vi "Decide next action (polarization-based).vi"(8 "error in (no error)":errorcluster, 10 "Seek positive polarization?":bool, 11 "Automatic Mode in":refnum<class "Automatic Mode.lvclass">) -> (0 "error out":errorcluster, 2 "Decision":T1, 3 "Automatic Mode out":refnum<class "Automatic Mode.lvclass">)   [LabVIEW 2015, in "Automatic Mode.lvclass"]
uses:
  Automatic Mode.lvclass
  Controller decision.ctl
  Automatic Mode.lvclass/Automatic Mode.ctl
  <vilib>/gmath/NI_Gmath.lvlib
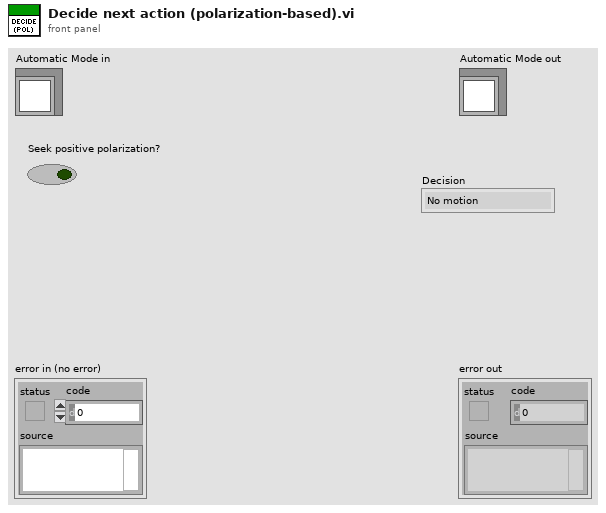
[diagram p1: front panel]
types:
  T1 = typedef "Controller decision.ctl" = enum16{"No motion", "Switch direction", "Keep current direction"}
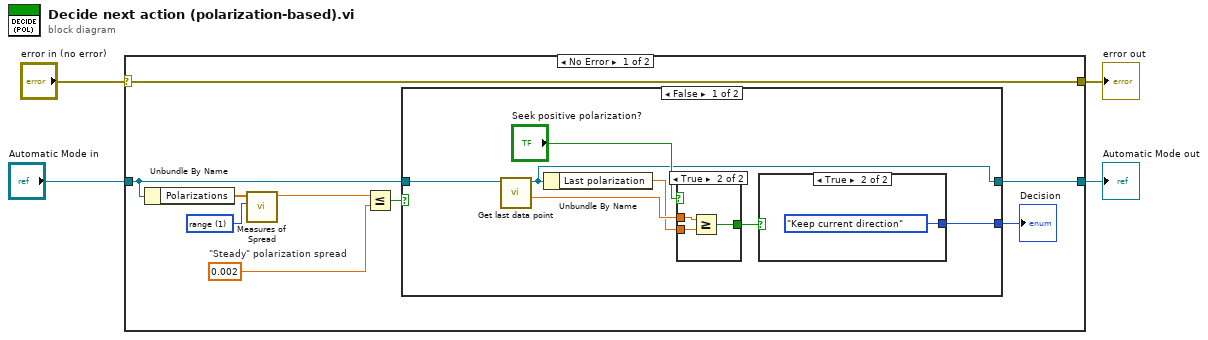
[diagram p0: block diagram]
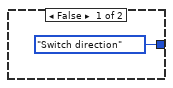
[diagram p2: hidden frame]
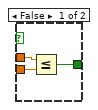
[diagram p3: hidden frame]
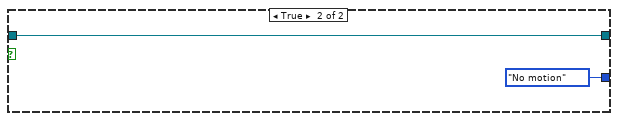
[diagram p4: hidden frame]
diagram:
  n1 = case shown="No Error" "error in (no error)" {
    selector: "error in (no error)" -> [w13 w32]
    tunnel: [w13 w32] -> w3
    tunnel: [w12 w31] -> w1
    tunnel: "Automatic Mode in" -> [w10 w31]
    frame No Error {
      w5 = 0.002  # "Steady" polarization spread
      w9 = 1 items=["standard deviation", "range", "mean absolute deviation", "interquartile range"] ("type")
      n2 = Unbundle By Name(w10) -> ("Polarizations"=w8:dbl[])
      n3 = call <vilib>:"Measures of Spread.vi"("type"=w9, "x array"=w8) -> ("spread value"=w7:dbl)  [unwired: 8 in, 1 out]
      n4 = Less Or Equal?(x=w7, y=w5) -> (x <= y?=w6:bool)
      n5 = case shown="False" w6 {
        tunnel: [w19 w29] -> w12
        tunnel: [w15 Controller_decision."No motion" ("Decision")] -> w11
        tunnel: w10 -> [w14 w29]
        frame False {
          n6 = call "Get last data point.vi"("Automatic Mode in"=w14) -> ("Polarization"=w18:dbl, "Automatic Mode out"=w19:refnum<class "Automatic Mode.lvclass">)  [unwired: 7 in, 2 out]
          n7 = Unbundle By Name(w19) -> ("Last polarization"=w17:dbl)
          n8 = case shown="True" "Seek positive polarization?" {
            tunnel: w18 -> [w25 w28]
            tunnel: w17 -> [w24 w27]
            tunnel: [w23 w26] -> w16
            frame False {
              n9 = Less Or Equal?(x=w25, y=w24) -> (x <= y?=w23:bool)
            }
            frame True {
              n10 = Greater Or Equal?(x=w28, y=w27) -> (x >= y?=w26:bool)
            }
          }
          n11 = case shown="True" w16 {
            tunnel: [Controller_decision."Switch direction" ("Decision") Controller_decision."Keep current direction" ("Decision")] -> w15
            frame False {
            }
            frame True {
            }
          }
        }
        frame True {
        }
      }
      "Decision" <- w11
    }
    frame Error {
    }
  }
  "error out" <- w3
  "Automatic Mode out" <- w1
